vi "标签打印.vi"(8 "错误输入（无错误）":errorcluster, 9 "流水号（3位）":string, 10 "班次":string, 11 "路径":path) -> (0 "error out":errorcluster caption="错误输出", 3 "Print":i32(ring) items=["btSuccess", "btTimeout", "btFailure"])   [LabVIEW 2012]
panel:
  in  "BarTender.IBtApplication":refnum<k7>
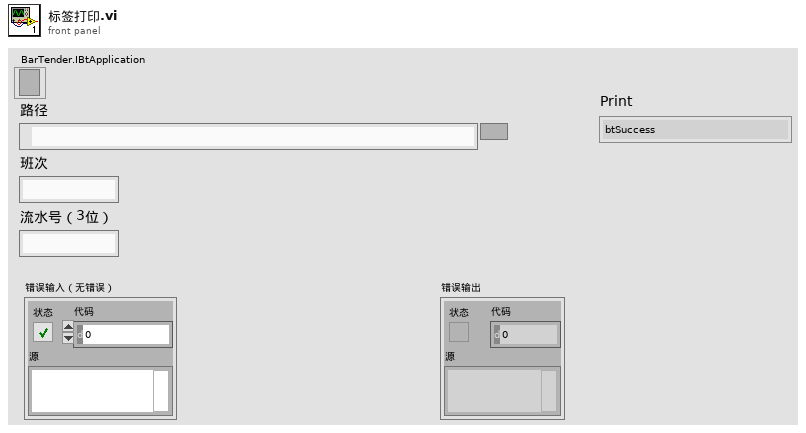
[diagram p1: front panel]
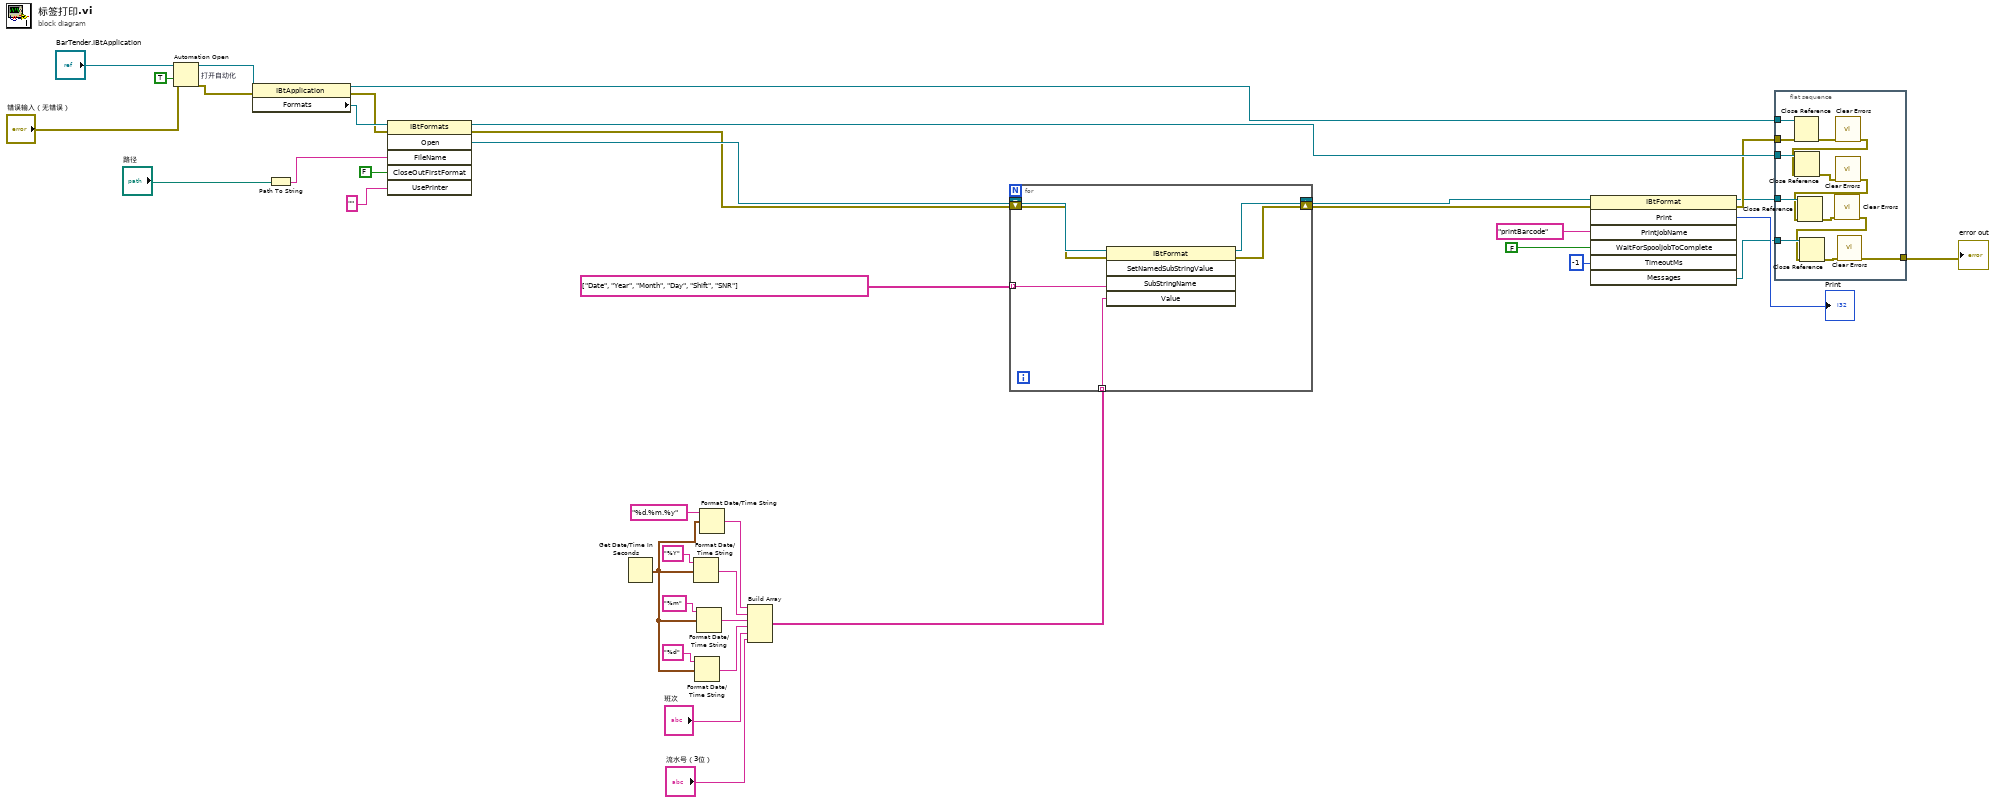
[diagram p0: block diagram]
diagram:
  n1 = Automation Open "打开自动化"(error in (no error)="错误输入（无错误）", Automation Refnum="BarTender.IBtApplication", 9:TRUE ("打开新实例（假）")) -> (Automation Refnum=w38:refnum<k7>, error out=w35:errorcluster)  [unwired: 1 in]
  n2 = property on="属性节点" class="IBtApplication"(reference=w38, error in=w35) -> (reference out=w33:refnum<k7>, error out=w34:errorcluster, "Formats"=w37:refnum<k7>)
  n3 = Path To String(path="路径") -> (string=w20:string)
  n4 = invoke on="调用节点" class="IBtFormats" method="Open"(reference=w37, error in=w34, "FileName"=w20, "CloseOutFirstFormat"=FALSE, "UsePrinter"="") -> (reference out=w32:refnum<k7>, error out=w21:errorcluster, "Open"=w22:refnum<k7>)  [unwired: 1 in, 3 out]
  n5 = Get Date/Time In Seconds() -> (seconds since 1Jan1904=w8:timestamp)
  n6 = Format Date/Time String(time format string (%c)="%Y" ("时间格式字符串(%c)"), seconds (now)=w8) -> (date/time string=w7:string)  [unwired: 1 in]
  n7 = Format Date/Time String(time format string (%c)="%d" ("时间格式字符串(%c)"), seconds (now)=w8) -> (date/time string=w5:string)  [unwired: 1 in]
  n8 = Format Date/Time String(time format string (%c)="%m" ("时间格式字符串(%c)"), seconds (now)=w8) -> (date/time string=w6:string)  [unwired: 1 in]
  n9 = Format Date/Time String(time format string (%c)="%d.%m.%y" ("时间格式字符串(%c)"), seconds (now)=w8) -> (date/time string=w12:string)  [unwired: 1 in]
  n10 = Build Array(w12, w7, w6, w5, "班次", "流水号（3位）") -> (w11:string[])
  n11 = for {
    shift-right: [w42] -> w15
    shift-left: w22 -> [w44]
    shift-right: [w41] -> w14
    shift-left: w21 -> [w43]
    tunnel: string[] ["Date", "Year", "Month", "Day", "Shift", "SNR"] -> [w40] mode=indexing
    tunnel: w11 -> [w39] mode=indexing
    n12 = invoke on="调用节点" class="IBtFormat" method="SetNamedSubStringValue"(reference=w44, error in=w43, "SubStringName"=w40, "Value"=w39) -> (reference out=w42:refnum<k7>, error out=w41:errorcluster)  [unwired: 1 in, 3 out]
  }
  n13 = invoke on="调用节点" class="IBtFormat" method="Print"(reference=w15, error in=w14, "PrintJobName"="printBarcode", "WaitForSpoolJobToComplete"=FALSE, "TimeoutMs"=-1) -> (reference out=w25:refnum<k7>, error out=w26:errorcluster, "Print"=→"Print":i32, "Messages"=w16:refnum<k7>)  [unwired: 2 in, 3 out]
  n14 = flat-sequence {
    tunnel: w33 -> [w57]
    tunnel: w32 -> [w56]
    tunnel: w26 -> [w55]
    tunnel: w25 -> [w54]
    tunnel: w16 -> [w47]
    tunnel: [w45] -> w1
    frame #0 {
      n15 = Close Reference(reference=w57, error in (no error)=w55) -> (error out=w50:errorcluster)
      n16 = call <vilib>:"Clear Errors.vi"("error in (no error)"=w50) -> ("error out"=w49:errorcluster)  [unwired: 5 in, 1 out]
      n17 = Close Reference(reference=w56, error in (no error)=w49) -> (error out=w52:errorcluster)
      n18 = call <vilib>:"Clear Errors.vi"("error in (no error)"=w52) -> ("error out"=w51:errorcluster)  [unwired: 5 in, 1 out]
      n19 = Close Reference(reference=w54, error in (no error)=w51) -> (error out=w53:errorcluster)
      n20 = call <vilib>:"Clear Errors.vi"("error in (no error)"=w53) -> ("error out"=w46:errorcluster)  [unwired: 5 in, 1 out]
      n21 = Close Reference(reference=w47, error in (no error)=w46) -> (error out=w48:errorcluster)
      n22 = call <vilib>:"Clear Errors.vi"("error in (no error)"=w48) -> ("error out"=w45:errorcluster)  [unwired: 5 in, 1 out]
    }
  }
  "error out" <- w1
